vi "preload default boot.vi"() -> (0 "PreLoad error":errorcluster)   [LabVIEW 2016]
doc: "This is the start up vi for the Lois program. It loads the files in the correct order."
panel:
  out "Front Panel Close":errorcluster
  out "BootFile error":errorcluster
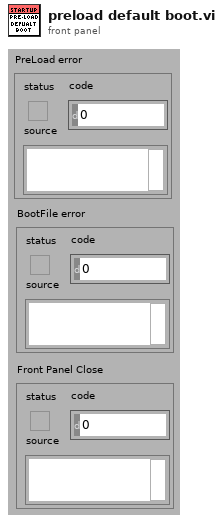
[diagram p1: front panel]
types:
  T1 = enum32{"Invalid", "Standard", "Closed", "Hidden", "Minimized", "Maximized"}
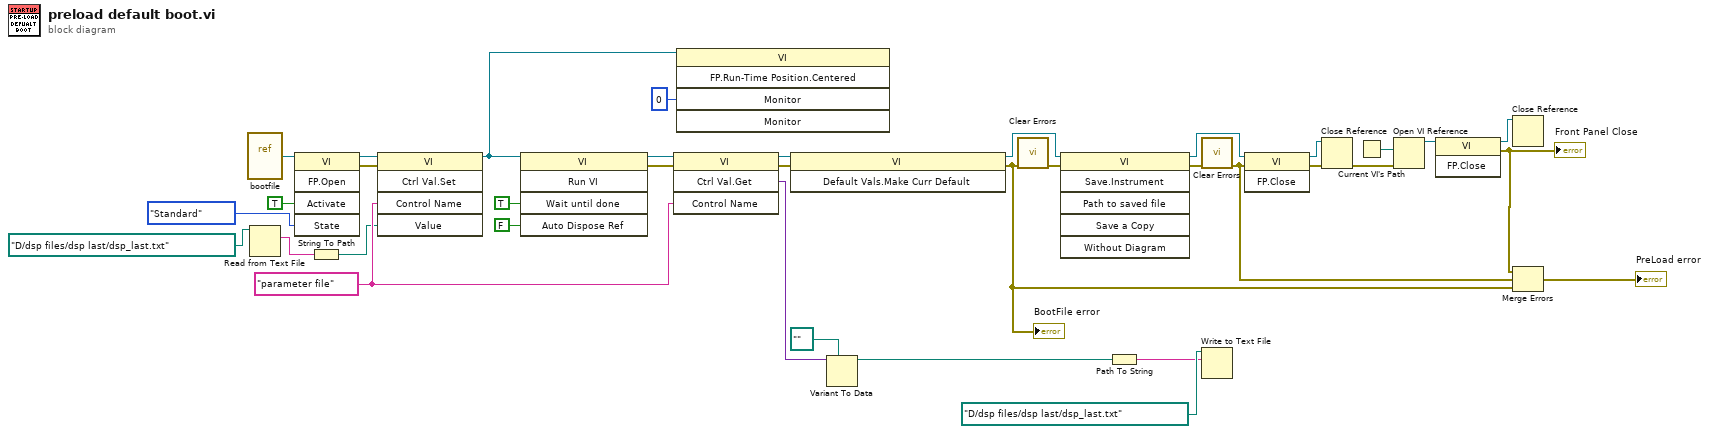
[diagram p0: block diagram]
diagram:
  w11 = "parameter file" ("Control Name")
  n1 = vi-ref "bootfile.vi"() -> (w32:refnum<vi>)
  n2 = Read from Text File(file (use dialog)=path "D:/dsp files/dsp last/dsp_last.txt") -> (text=w7:string)  [unwired: 3 in, 3 out]
  n3 = invoke class="VI" method="FP.Open"(reference=w32, "Activate"=TRUE ("Activate?"), "State"=T1."Standard") -> (reference out=w13:refnum<vi>, error out=w12:errorcluster)  [unwired: 2 in, 3 out]
  n4 = String To Path(string=w7) -> (path=w6:path)
  n5 = invoke class="VI" method="Ctrl Val.Set"(reference=w13, error in=w12, "Control Name"=w11, "Value"=w6) -> (reference out=w5:refnum<vi>)  [unwired: 1 in, 4 out]
  n6 = invoke class="VI" method="Run VI"(reference=w5, "Wait until done"=TRUE ("Wait Until Done"), "Auto Dispose Ref"=FALSE ("Auto Dispose Reference")) -> (reference out=w19:refnum<vi>, error out=w20:errorcluster)  [unwired: 2 in, 3 out]
  n7 = invoke class="VI" method="Ctrl Val.Get"(reference=w19, error in=w20, "Control Name"=w11) -> (reference out=w18:refnum<vi>, error out=w17:errorcluster, "Get Control Value Variant"=w16:variant)  [unwired: 1 in, 1 out]
  n8 = invoke class="VI" method="FP.Run-Time Position.Centered"(reference=w5, "Monitor"=i16 0) -> ()  [unwired: 3 in, 5 out]
  n9 = invoke class="VI" method="Default Vals.Make Curr Default"(reference=w18, error in=w17) -> (reference out=w31:refnum<vi>, error out=w3:errorcluster)  [unwired: 1 in, 1 out]
  "BootFile error" <- w3
  n10 = Variant To Data(type=path "" ("file (use dialog)"), Variant=w16) -> (data=w9:path)  [unwired: 1 in, 1 out]
  n11 = call <vilib>:"Clear Errors.vi"("error in (no error)"=w3) -> ("error out"=w25:errorcluster)  [unwired: 5 in, 1 out]
  n12 = invoke class="VI" method="Save.Instrument"(reference=w31, error in=w25) -> (reference out=w30:refnum<vi>, error out=w24:errorcluster)  [unwired: 4 in, 4 out]
  n13 = Path To String(path=w9) -> (string=w8:string)
  n14 = call <vilib>:"Clear Errors.vi"("error in (no error)"=w24) -> ("error out"=w23:errorcluster)  [unwired: 5 in, 1 out]
  n15 = Write to Text File(file (use dialog)=path "D:/dsp files/dsp last/dsp_last.txt", text=w8) -> ()  [unwired: 2 in, 3 out]
  n16 = invoke class="VI" method="FP.Close"(reference=w30, error in=w23) -> (reference out=w35:refnum<vi>, error out=w27:errorcluster)  [unwired: 1 in, 1 out]
  n17 = Close Reference(reference=w35, error in (no error)=w27) -> (error out=w28:errorcluster)
  n18 = Current VI's Path() -> (path=w29:path)
  n19 = Open VI Reference(vi path=w29, error in (no error)=w28) -> (vi reference=w22:refnum<vi>)  [unwired: 4 in, 1 out]
  n20 = invoke class="VI" method="FP.Close"(reference=w22) -> (reference out=w26:refnum<vi>, error out=w2:errorcluster)  [unwired: 2 in, 1 out]
  "Front Panel Close" <- w2
  n21 = Close Reference(reference=w26) -> ()  [unwired: 1 in, 1 out]
  n22 = Merge Errors(w2, w23, w3) -> (→"PreLoad error":errorcluster)
